vi "publish -- set -- 5.vi"(8 "request event":refnum<user-event>, 9 "response event":refnum<user-event>, 10 "number":dbl=1000.0 format="%#_10f") -> ()   [LabVIEW 2018]
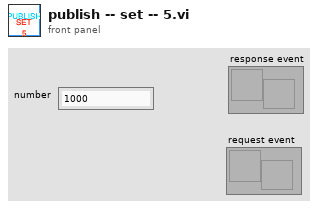
[diagram p1: front panel]
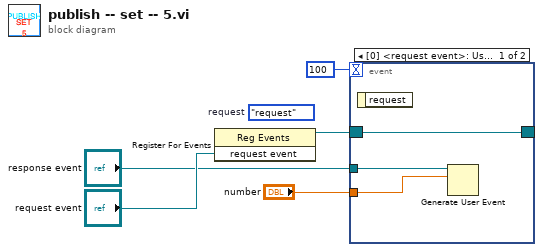
[diagram p0: block diagram]
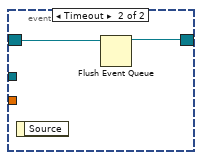
[diagram p2: hidden frame]
diagram:
  (unwired) enum16{"request"}."request"  # request
  n1 = register-events("request event") -> (reference out=w5:refnum<event-registration>)  [unwired: 2 in, 1 out]
  n2 = event shown="[0] <request event>: User Event" {
    selector: w5 -> [w8 w10]
    dyn-events: [w8 w9] -> _
    timeout: 100 -> [_ _]
    tunnel: "response event" -> [w7 _]
    tunnel: "number" -> [w6 _]
    event User Event {
      n3 = event-data() -> ()  [unwired: 1 in, 1 out]
      n4 = Generate User Event(user event=w7, event data cluster=w6) -> ()  [unwired: 2 in, 2 out]
    }
    event Timeout {
      n5 = event-data() -> ()  [unwired: 1 in, 1 out]
      n6 = Flush Event Queue(0:w10) -> (8:w9:refnum<event-registration>)  [unwired: 5 in, 2 out]
    }
  }
